vi "BrokenWhiteNoise Modifed.vi"() -> ()   [LabVIEW 2014]
uses:
  <vilib>/DAQmx/create/channels.llb/DAQmx Create Channel (AO-Voltage-Basic).vi
  <vilib>/DAQmx/configure/timing.llb/DAQmx Timing (Sample Clock).vi
  <vilib>/DAQmx/create/channels.llb/DAQmx Create Channel (AI-Voltage-Basic).vi
  <vilib>/DAQmx/write.llb/DAQmx Write (Analog Wfm 1Chan NSamp).vi
  <vilib>/DAQmx/read.llb/DAQmx Read (Analog Wfm 1Chan NSamp).vi
  <vilib>/measure/NI_MABase.lvlib
panel:
  in  "samples per channel":i32=1000
  out "Waveform Graph 2":waveform(dbl)(graph)
  out "?":errorcluster
  out "number of samples written per channel":u32=5000
  in  "Sample Rate AO":dbl=20000.0
  in  "Max Voltage AO":dbl=5.0
  in  "Min Voltage AO":dbl=-5.0
  in  "Physical Channel(s)":tag="Dev1/ao0"
  out "Waveform Graph":waveform(dbl)(graph)={"t0"=timestamp(0 s since 1904-01-01), "dt"=5e-05, "Y"=array[5000 elements]}
  out "Iterations":i32=108
  in  "Stop":bool
  out "White noise":errorcluster
  # "Analog output"
  # "Analog input"
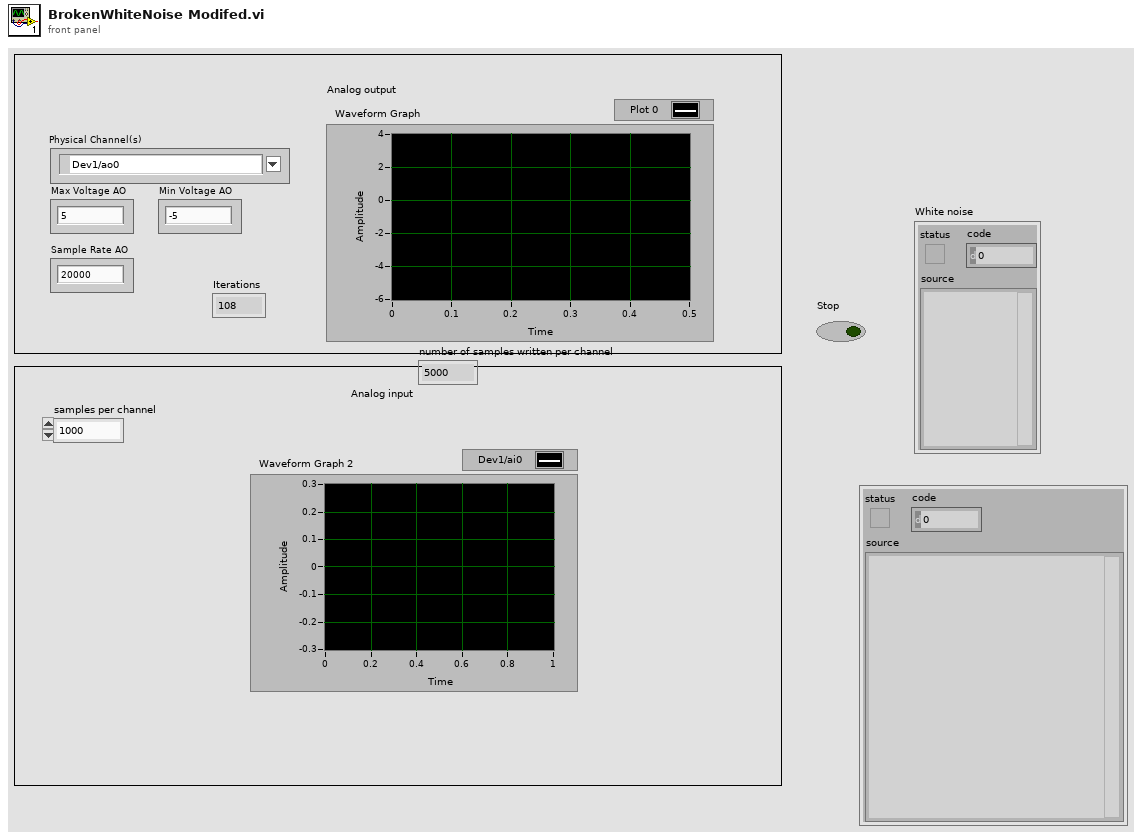
[diagram p1: front panel]
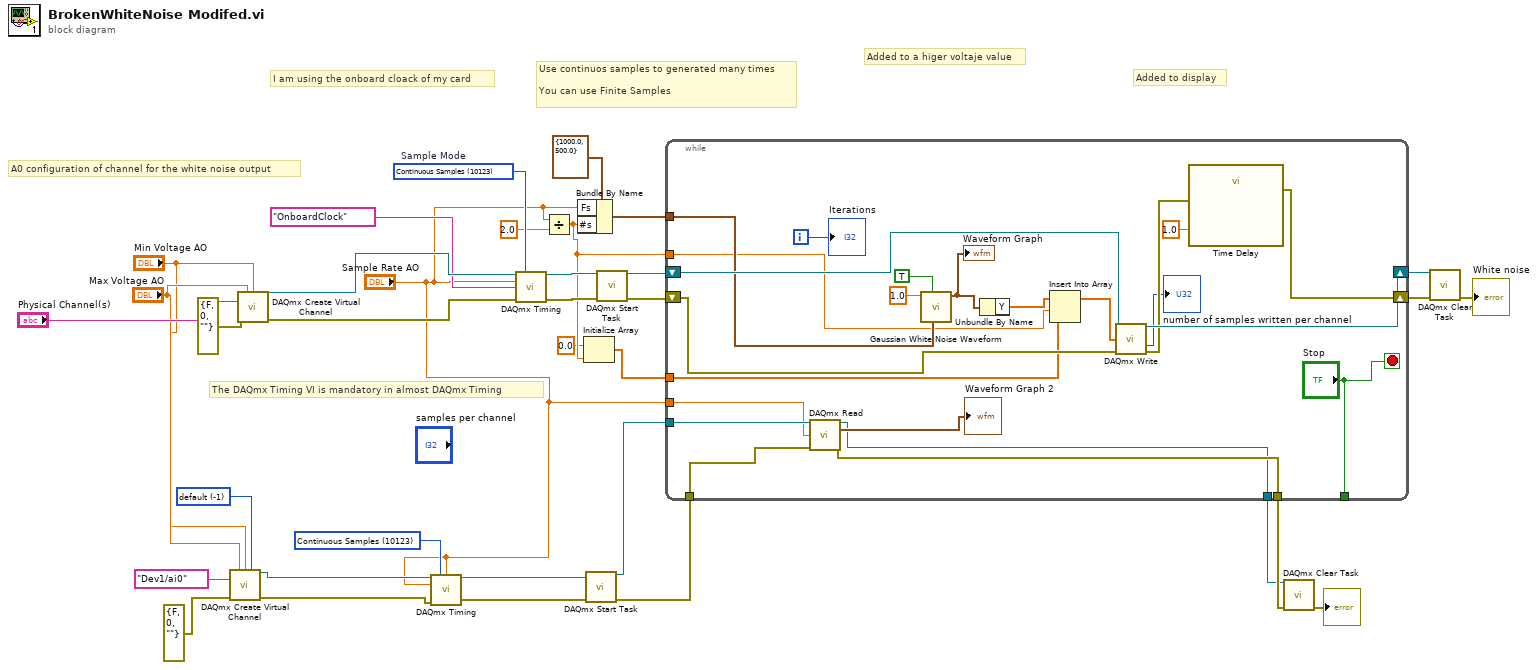
[diagram p0: block diagram]
diagram:
  w16 = 10123 items=["Finite Samples"=10178, "Continuous Samples"=10123, "Hardware Timed Single Point"=12522] ("sample mode")
  w18 = -1 items=["default"=-1, "RSE"=10083, "NRSE"=10078, "Differential"=10106, "Pseudodifferential"=12529] ("input terminal configuration")
  w33 = 10123 items=["Finite Samples"=10178, "Continuous Samples"=10123, "Hardware Timed Single Point"=12522]  # Sample Mode
  # "Use continuos samples to generated many times\n\nYou can use Finite Samples"
  # "Added to a higer voltaje value"
  # "Added to display"
  # "I am using the onboard cloack of my card"
  # "The DAQmx Timing VI is mandatory in almost DAQmx Timing"
  # "A0 configuration of channel for the white noise output"
  n1 = call-poly <vilib>:"DAQmx Create Virtual Channel.vi"("maximum value"="Max Voltage AO", "minimum value"="Min Voltage AO", "input terminal configuration"=w18, "physical channels"=tag "Dev1/ai0", "error in"=errorcluster {"status"=FALSE, "code"=0, "source"=""}) -> ("task out"=w22:refnum<k21>, "error out"=w19:errorcluster)  [unwired: 9 in]
  n2 = call-poly <vilib>:"DAQmx Create Virtual Channel.vi"("maximum value"="Max Voltage AO", "minimum value"="Min Voltage AO", "physical channels"="Physical Channel(s)", "error in"=errorcluster {"status"=FALSE, "code"=0, "source"=""}) -> ("task out"=w31:refnum<k21>, "error out"=w32:errorcluster)  [unwired: 10 in]
  n3 = call-poly <vilib>:"DAQmx Timing.vi"("task/channels in"=w22, "sample mode"=w16, "samples per channel"="Sample Rate AO", "rate"="Sample Rate AO", "error in"=w19) -> ("task out"=w21:refnum<k21>, "error out"=w20:errorcluster)  [unwired: 9 in]
  n4 = call-poly <vilib>:"DAQmx Timing.vi"("task/channels in"=w31, "sample mode"=w33, "rate"="Sample Rate AO", "source"=tag "OnboardClock", "error in"=w32) -> ("task out"=w26:refnum<k21>, "error out"=w28:errorcluster)  [unwired: 9 in]
  n5 = Divide(x="Sample Rate AO", y=2.0) -> (x/y=w4:dbl)
  n6 = Bundle By Name(cluster=cluster{"Fs":dbl, "#s":dbl} {"Fs"=1000.0, "#s"=500.0} ("sampling info"), "Fs"="Sample Rate AO", "#s"=w4) -> (w5:cluster{"Fs":dbl, "#s":dbl})
  n7 = Initialize Array(0.0 ("element"), w4) -> (w3:dbl[])
  n8 = call <vilib>:"DAQmx Start Task.vi"("task/channels in"=w21, "error in"=w20) -> ("task out"=w11:refnum<k21>, "error out"=w10:errorcluster)  [unwired: 12 in]
  n9 = call <vilib>:"DAQmx Start Task.vi"("task/channels in"=w26, "error in"=w28) -> ("task out"=w25:refnum<k21>, "error out"=w27:errorcluster)  [unwired: 12 in]
  n10 = while {
    shift-right: [w56] -> w34
    shift-left: w25 -> [w58]
    shift-right: [w50] -> w23
    shift-left: w27 -> [w57]
    tunnel: ["Stop"] -> _
    tunnel: w11 -> [w45]
    tunnel: w10 -> [w44]
    tunnel: [w43] -> w9
    tunnel: [w42] -> w8
    tunnel: "Sample Rate AO" -> [w41]
    tunnel: w5 -> [w40]
    tunnel: w4 -> [w38]
    tunnel: w3 -> [w37]
    i -> [w55]
    stop <- "Stop" stop-if-true
    n11 = call-poly <vilib>:"DAQmx Read.vi"("task/channels in"=w45, "number of samples per channel"=w41, "error in"=w44) -> ("task out"=w42:refnum<k21>, "data"=→"Waveform Graph 2":waveform(dbl), "error out"=w43:errorcluster)  [unwired: 10 in]
    n12 = call <vilib>:"Gaussian White Noise Waveform.vi"("sampling info"=w40, "reset signal"=TRUE, "standard deviation"=1.0) -> ("signal out"=w48:waveform(dbl))  [unwired: 7 in, 1 out]
    "Waveform Graph" <- w48
    n13 = Unbundle By Name(w48) -> ("Y"=w39:dbl[])
    n14 = Insert Into Array(array=w39, index=w38, new element=w37) -> (w36:dbl[])
    n15 = call-poly <vilib>:"DAQmx Write.vi"("task/channels in"=w58, "data"=w36, "error in"=w57) -> ("task out"=w56:refnum<k21>, "number of samples written per channel"=→"number of samples written per channel":u32, "error out"=w51:errorcluster)  [unwired: 10 in]
    n16 = call "Time Delay"("error in (no error)"=w51, "Delay Time (s)"=1.0) -> ("error out"=w50:errorcluster)  [unwired: 9 in]
    "Iterations" <- w55
  }
  n17 = call <vilib>:"DAQmx Clear Task.vi"("task in"=w8, "error in"=w9) -> ("error out"=→"?":errorcluster)  [unwired: 13 in]
  n18 = call <vilib>:"DAQmx Clear Task.vi"("task in"=w34, "error in"=w23) -> ("error out"=→"White noise":errorcluster)  [unwired: 13 in]
